vi "3.11-Calculate Max Steering Angle.vi"(2 "Left Data":cluster{"Left Angle":dbl, "Left Magnitude":dbl}, 3 "Right Data":T1) -> (0 "Left Max Turn":dbl, 1 "Right Max Turn":dbl)   [LabVIEW 2010]
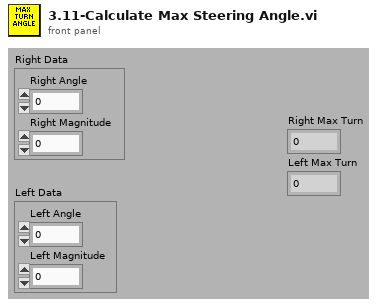
[diagram p1: front panel]
types:
  T1 = cluster{"Right Angle":dbl, "Right Magnitude":dbl}
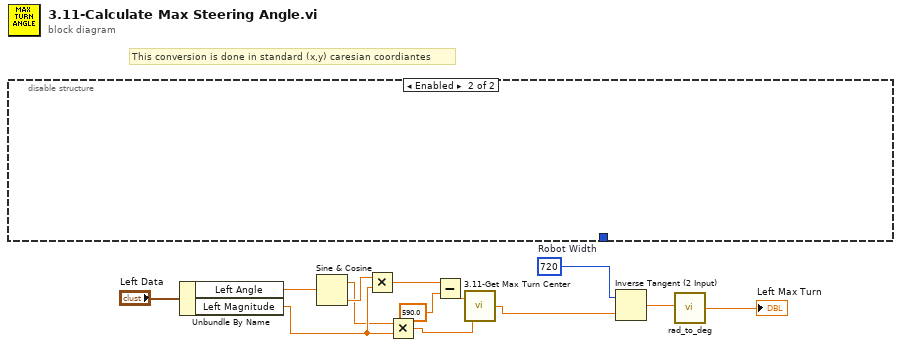
[diagram p0: block diagram]
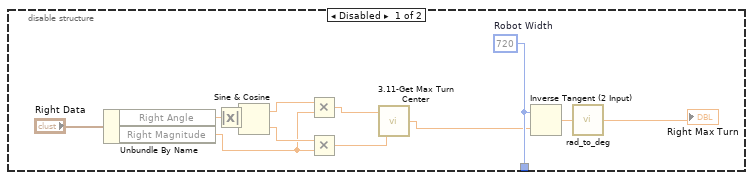
[diagram p2: hidden frame]
diagram:
  w8 = 720  # Robot Width
  # "This conversion is done in standard (x,y) caresian coordiantes"
  n1 = disable-structure shown="Enabled" {
    disable-tunnel: [w20 _] -> _
    frame Disabled {
      w20 = 720  # Robot Width
      n2 = Unbundle By Name("Right Data") -> ("Right Angle"=w17:dbl, "Right Magnitude"=w22:dbl)
      n3 = Absolute Value(x=w17) -> (abs(x)=w16:dbl)
      n4 = Sine & Cosine(0:w16) -> (1:w23:dbl, 2:w24:dbl)
      n5 = Multiply(x=w23, y=w22) -> (x*y=w15:dbl)
      n6 = Multiply(x=w24, y=w22) -> (x*y=w21:dbl)
      n7 = call "3.11-Get Max Turn Center.vi"("X (mm)"=w21, "Y (mm)"=w15) -> ("Start Turn Angle"=w14:dbl)
      n8 = Inverse Tangent (2 Input)(1:w14, 2:w20) -> (0:w19:dbl)
      n9 = call "rad_to_deg.vi"("Radians"=w19) -> ("Degrees"=→"Right Max Turn":dbl)
    }
    frame Enabled {
    }
  }
  n10 = Unbundle By Name("Left Data") -> ("Left Angle"=w1:dbl, "Left Magnitude"=w12:dbl)
  n11 = Sine & Cosine(0:w1) -> (1:w2:dbl, 2:w3:dbl)
  n12 = Multiply(x=w3, y=w12) -> (x*y=w4:dbl)
  n13 = Multiply(x=w2, y=w12) -> (x*y=w7:dbl)
  n14 = Subtract(x=w4, y=590.0) -> (x-y=w6:dbl)
  n15 = call "3.11-Get Max Turn Center.vi"("X (mm)"=w7, "Y (mm)"=w6) -> ("Start Turn Angle"=w10:dbl)
  n16 = Inverse Tangent (2 Input)(1:w10, 2:w8) -> (0:w11:dbl)
  n17 = call "rad_to_deg.vi"("Radians"=w11) -> ("Degrees"=→"Left Max Turn":dbl)
